vi "InitTurret.vi"   [LabVIEW 2020]
doc: "This VI initializes devices related to the turret subsystem."
uses:
  <vilib>/Rock Robotics/WPI/ThirdParty/Phoenix-LabVIEW/Motor Controller/Controls/CTRE_Phoenix_MotorControl_TalonFXInvertType.ctl
  <vilib>/Rock Robotics/WPI/ThirdParty/Phoenix-LabVIEW/Motor Controller/Controls/CTRE_Phoenix_MotorControl_NeutralMode.ctl
  <vilib>/Rock Robotics/WPI/ThirdParty/Phoenix-LabVIEW/Motor Controller/Controls/CTRE_Phoenix_MotorControl_SupplyCurrentLimitConfiguration.ctl
  <vilib>/Rock Robotics/WPI/ThirdParty/Phoenix-LabVIEW/Motor Controller/Controls/CTRE_Phoenix_MotorControl_FeedbackDevice_TalonFX.ctl
  <vilib>/Rock Robotics/WPI/ThirdParty/Phoenix-LabVIEW/Motor Controller/Controls/CTRE_Phoenix_MotorControl_LimitSwitchSource_Local.ctl
  <vilib>/Rock Robotics/WPI/ThirdParty/Phoenix-LabVIEW/Motor Controller/Controls/CTRE_Phoenix_MotorControl_LimitSwitchNormal.ctl
  refnumbers.vi
  robotconstants.vi
types:
  T1 = typedef "CTRE_Phoenix_MotorControl_LimitSwitchNormal.ctl" = enum16{"Normally Open", "Normally Closed", "Disabled"}
  T2 = typedef "CTRE_Phoenix_MotorControl_LimitSwitchSource_Local.ctl" = enum16{"Feedback Connector", "Remote Talon SRX", "Remote CANifier", "Deactivated"}
  T3 = typedef "CTRE_Phoenix_MotorControl_FeedbackDevice_TalonFX.ctl" = i8
  T4 = typedef "CTRE_Phoenix_MotorControl_SupplyCurrentLimitConfiguration.ctl" = cluster{"Enable?":bool, "Current Limit":dbl, "Threshold Current":dbl, "Threshold Time":dbl}
  T5 = typedef "CTRE_Phoenix_MotorControl_NeutralMode.ctl" = enum8{"EEPROMSetting", "Override to Coast", "Override to Brake"}
  T6 = typedef "CTRE_Phoenix_MotorControl_TalonFXInvertType.ctl" = enum16{"Counter-Clockwise", "Clockwise"}
  T7 = typedef "WPI_MotorControlDeviceRef.ctl" = cluster{"DeviceStatus":errorcluster, "Type":T8, "PWM":cluster{"PWM Channel":T9, "DeadBand":T10}, "CAN":cluster{"Device Number":u8, "SetOutput VI Ref":variant, "GetOutput VI Ref":variant, "Enable VI Ref":variant, "Disable VI Ref":variant, "Data":variant}, "Invert":bool, "DIO PWM":cluster{"PWM \"Enable\" Channel":T9, "DIOChannel":T11, "PWM Rate":dbl}}
  T8 = typedef "WPI_MotorControlType.ctl" = enum16{"PWM", "CAN", "DIO PWM"}
  T9 = typedef "FPGA_DIOPWMChannel.ctl" = enum8{"PWM 0", "PWM 1", "PWM 2", "PWM 3", "PWM 4", "PWM 5", "PWM 6", "PWM 7", "PWM 8", "PWM 9", "PWM MXP 0", "PWM MXP 1", "PWM MXP 2", "PWM MXP 3", "PWM MXP 4", "PWM MXP 5", "PWM MXP 6", "PWM MXP 7", "PWM MXP 8", "PWM MXP 9", "Invalid"}
  T10 = typedef "WPI_PWMDeadband.ctl" = cluster{"Name":string, "maxPositivePwm":i32, "minPositivePwm":i32, "centerPwm":i32, "maxNegativePwm":i32, "minNegativePwm":i32, "angularRange":u16}
  T11 = typedef "FPGA_DIOChannel.ctl" = enum8{"DIO 0", "DIO 1", "DIO 2", "DIO 3", "DIO 4", "DIO 5", "DIO 6", "DIO 7", "DIO 8", "DIO 9", "DIO MXP 0", "DIO MXP 1", "DIO MXP 2", "DIO MXP 3", "DIO MXP 4", "DIO MXP 5", "DIO MXP 6", "DIO MXP 7", "DIO MXP 8", "DIO MXP 9", "DIO MXP 10", "DIO MXP 11", "DIO MXP 12", "DIO MXP 13", "DIO MXP 14", "DIO MXP 15", "SPI Port CS1", "SPI Port CS2", "SPI Port CS3", "SPI Port MISO", "SPI Port MOSI", "Invalid"}
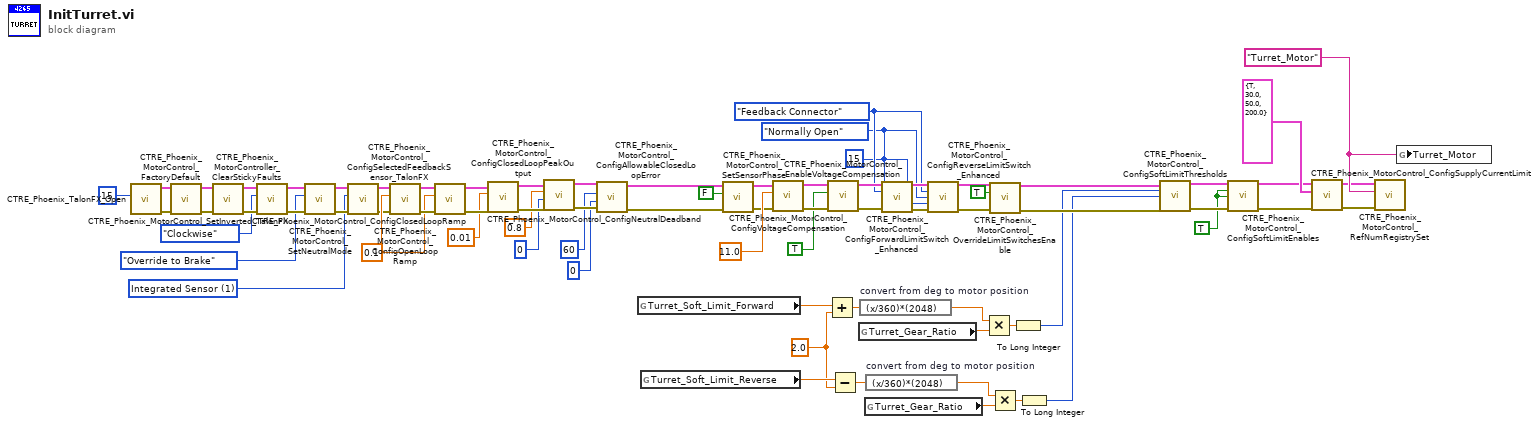
[diagram p0: block diagram]
diagram:
  w17 = 2.0 ("y")
  w24 = TRUE ("Forward Soft Limit Enable")
  w43 = 15 ("deviceID")
  w44 = CTRE_Phoenix_MotorControl_LimitSwitchNormal."Normally Open" ("NormallyOpenOrClosed")
  w45 = CTRE_Phoenix_MotorControl_LimitSwitchSource_Local."Feedback Connector" ("Limit Switch Source")
  w49 = T3 1 items=["Integrated Sensor"=1, "Sensor Sum (S0 + S1)"=9, "Sensor Difference (D0 - D1)"=10, "Remote Source 0"=11, "Remote Source 1"=12, "None"=14, "Software Emulated"=15] ("Talon FX Feedback Device")
  w55 = 0.1 ("secondsFromNeutralToFull")
  w71 = "Turret_Motor" ("refnum name")
  n1 = call <vilib>:"CTRE_Phoenix_TalonFX_Open.vi"("Device Number"=u8 15 ("Drive 4L")) -> ("error out"=w60:errorcluster, "PhoenixMotorControlDevRef"=w67:T7)  [unwired: 9 in]
  n2 = call <vilib>:"CTRE_Phoenix_MotorControl_FactoryDefault.vi"("error in"=w60, "PhoenixMotorControlDevRef"=w67) -> ("error out"=w63:errorcluster, "PhoenixMotorControlDevRef"=w64:T7)  [unwired: 8 in]
  n3 = call <vilib>:"CTRE_Phoenix_MotorController_ClearStickyFaults.vi"("error in"=w63, "PhoenixMotorControlDevRef"=w64) -> ("error out"=w62:errorcluster, "PhoenixMotorControlDevRef"=w61:T7)  [unwired: 8 in]
  n4 = call <vilib>:"CTRE_Phoenix_MotorControl_SetInverted_TalonFX.vi"("error in (no error)"=w62, "Invert Type"=CTRE_Phoenix_MotorControl_TalonFXInvertType."Clockwise", "PhoenixMotorControlDevRef"=w61) -> ("error out"=w72:errorcluster, "PhoenixMotorControlDevRef"=w73:T7)  [unwired: 7 in]
  n5 = call <vilib>:"CTRE_Phoenix_MotorControl_SetNeutralMode.vi"("error in (no error)"=w72, "Motor Control Neutral Mode"=CTRE_Phoenix_MotorControl_NeutralMode."Override to Brake", "PhoenixMotorControlDevRef"=w73) -> ("error out"=w58:errorcluster, "PhoenixMotorControlDevRef"=w59:T7)  [unwired: 7 in]
  n6 = call <vilib>:"CTRE_Phoenix_MotorControl_ConfigSelectedFeedbackSensor_TalonFX.vi"("error in (no error)"=w58, "Talon FX Feedback Device"=w49, "PhoenixMotorControlDevRef"=w59) -> ("error out"=w37:errorcluster, "PhoenixMotorControlDevRef"=w38:T7)  [unwired: 7 in]
  n7 = call <vilib>:"CTRE_Phoenix_MotorControl_ConfigOpenLoopRamp.vi"("error in (no error)"=w37, "secondsFromNeutralToFull"=w55, "PhoenixMotorControlDevRef"=w38) -> ("error out"=w65:errorcluster, "PhoenixMotorControlDevRef"=w66:T7)  [unwired: 7 in]
  n8 = call <vilib>:"CTRE_Phoenix_MotorControl_ConfigClosedLoopRamp.vi"("error in (no error)"=w65, "secondsFromNeutralToFull"=w55, "PhoenixMotorControlDevRef"=w66) -> ("error out"=w32:errorcluster, "PhoenixMotorControlDevRef"=w33:T7)  [unwired: 7 in]
  n9 = call <vilib>:"CTRE_Phoenix_MotorControl_ConfigNeutralDeadband.vi"("error in (no error)"=w32, "Percent Deadband"=0.01, "PhoenixMotorControlDevRef"=w33) -> ("error out"=w10:errorcluster, "PhoenixMotorControlDevRef"=w9:T7)  [unwired: 7 in]
  n10 = call <vilib>:"CTRE_Phoenix_MotorControl_ConfigClosedLoopPeakOutput.vi"("error in (no error)"=w10, "slotIdx"=0, "peakOutput"=0.8, "PhoenixMotorControlDevRef"=w9) -> ("error out"=w4:errorcluster, "PhoenixMotorControlDevRef"=w6:T7)  [unwired: 6 in]
  n11 = call <vilib>:"CTRE_Phoenix_MotorControl_ConfigAllowableClosedLoopError.vi"("error in (no error)"=w4, "slotIdx"=u32 0, "allowableClosedLoopError"=60, "PhoenixMotorControlDevRef"=w6) -> ("error out"=w3:errorcluster, "PhoenixMotorControlDevRef"=w5:T7)  [unwired: 6 in]
  n12 = global read "robotconstants.vi" "Turret_Soft_Limit_Forward"() -> (w23:dbl)
  n13 = global read "robotconstants.vi" "Turret_Soft_Limit_Reverse"() -> (w22:dbl)
  n14 = call <vilib>:"CTRE_Phoenix_MotorControl_SetSensorPhase.vi"("error in (no error)"=w3, "PhaseSensor"=FALSE, "PhoenixMotorControlDevRef"=w5) -> ("error out"=w34:errorcluster, "PhoenixMotorControlDevRef"=w35:T7)  [unwired: 7 in]
  n15 = call <vilib>:"CTRE_Phoenix_MotorControl_ConfigVoltageCompensation.vi"("error in (no error)"=w34, "Saturation Voltage"=11.0, "PhoenixMotorControlDevRef"=w35) -> ("error out"=w53:errorcluster, "PhoenixMotorControlDevRef"=w54:T7)  [unwired: 7 in]
  n16 = Add(x=w23, y=w17) -> (x+y=w18:dbl)
  n17 = call <vilib>:"CTRE_Phoenix_MotorControl_EnableVoltageCompensation.vi"("error in (no error)"=w53, "Enable Voltage Compensation?"=TRUE, "PhoenixMotorControlDevRef"=w54) -> ("error out"=w40:errorcluster, "PhoenixMotorControlDevRef"=w46:T7)  [unwired: 7 in]
  n18 = Subtract(x=w22, y=w17) -> (x-y=w13:dbl)
  n19 = global read "robotconstants.vi" "Turret_Gear_Ratio"() -> (w19:dbl)
  n20 = expression code="(x/360)*(2048)" "convert from deg to motor position"(w18) -> (w21:dbl)
  n21 = global read "robotconstants.vi" "Turret_Gear_Ratio"() -> (w14:dbl)
  n22 = expression code="(x/360)*(2048)" "convert from deg to motor position"(w13) -> (w16:dbl)
  n23 = call <vilib>:"CTRE_Phoenix_MotorControl_ConfigForwardLimitSwitch_Enhanced.vi"("PhoenixMotorControlDevRef"=w46, "Limit Switch Source"=w45, "NormallyOpenOrClosed"=w44, "deviceID"=w43, "error in (no error)"=w40) -> ("PhoenixMotorControlDevRef"=w48:T7, "error out"=w47:errorcluster)  [unwired: 9 in]
  n24 = call <vilib>:"CTRE_Phoenix_MotorControl_ConfigReverseLimitSwitch_Enhanced.vi"("PhoenixMotorControlDevRef"=w48, "Limit Switch Source"=w45, "NormallyOpenOrClosed"=w44, "deviceID"=w43, "error in (no error)"=w47) -> ("PhoenixMotorControlDevRef"=w42:T7, "error out"=w39:errorcluster)  [unwired: 9 in]
  n25 = Multiply(x=w21, y=w19) -> (x*y=w20:dbl)
  n26 = call <vilib>:"CTRE_Phoenix_MotorControl_OverrideLimitSwitchesEnable.vi"("PhoenixMotorControlDevRef"=w42, "Override Limit Switch Enable?"=TRUE, "error in (no error)"=w39) -> ("PhoenixMotorControlDevRef"=w30:T7, "error out"=w29:errorcluster)  [unwired: 11 in]
  n27 = Multiply(x=w16, y=w14) -> (x*y=w15:dbl)
  n28 = To Long Integer(number=w20) -> (32bit integer=w12:i32)
  n29 = To Long Integer(number=w15) -> (32bit integer=w11:i32)
  n30 = call <vilib>:"CTRE_Phoenix_MotorControl_ConfigSoftLimitThresholds.vi"("PhoenixMotorControlDevRef"=w30, "Forward Soft Limit"=w12, "Reverse Soft Limit"=w11, "error in (no error)"=w29) -> ("PhoenixMotorControlDevRef"=w27:T7, "error out"=w28:errorcluster)  [unwired: 10 in]
  n31 = call <vilib>:"CTRE_Phoenix_MotorControl_ConfigSoftLimitEnables.vi"("PhoenixMotorControlDevRef"=w27, "Forward Soft Limit Enable"=w24, "Reverse Soft Limit Enable"=w24, "error in (no error)"=w28) -> ("PhoenixMotorControlDevRef"=w26:T7, "error out"=w25:errorcluster)  [unwired: 10 in]
  n32 = call <vilib>:"CTRE_Phoenix_MotorControl_ConfigSupplyCurrentLimit.vi"("error in (no error)"=w25, "Supply Current Limit Configuration"=T4 {"Enable?"=TRUE, "Current Limit"=30.0, "Threshold Current"=50.0, "Threshold Time"=200.0}, "PhoenixMotorControlDevRef"=w26) -> ("error out"=w69:errorcluster, "PhoenixMotorControlDevRef"=w70:T7)  [unwired: 7 in]
  n33 = call <vilib>:"CTRE_Phoenix_MotorControl_RefNumRegistrySet.vi"("error in (no error)"=w69, "refnum name"=w71, "PhoenixMotorControlDevRef"=w70) -> ()  [unwired: 7 in, 2 out]
  n34 = global write "refnumbers.vi" "Turret_Motor"(w71) -> ()
